vi "SubVI_counter_PM.VI"(2 "DeviceIndex":i32, 3 "Ch1 parameters":T1={"Ch1 Offs"=0, "Ch1 TRG Edge"=0, "Ch1 TRG Lvl"=-50} {"Ch1 TRG Lvl" min=-1200 max=1200 step=10; "Ch1 TRG Edge" min=0 max=1; "Ch1 Offs" min=-99999 max=99999 step=1}, 4 "Acq.Time (ms)":i32=10000 min=1 max=3600000 step=100) -> (0 "FiFoOverrun":bool, 1 "Counts":i32)   [LabVIEW 2013]
uses:
  th260lib.dll
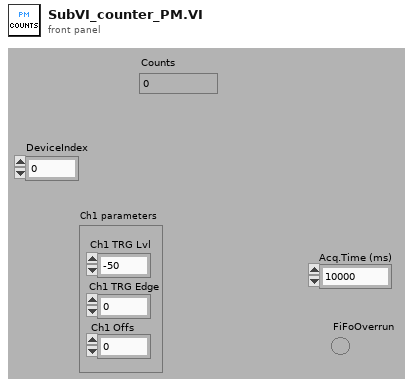
[diagram p1: front panel]
types:
  T1 = cluster{"Ch1 Offs":i32, "Ch1 TRG Edge":i32, "Ch1 TRG Lvl":i32}
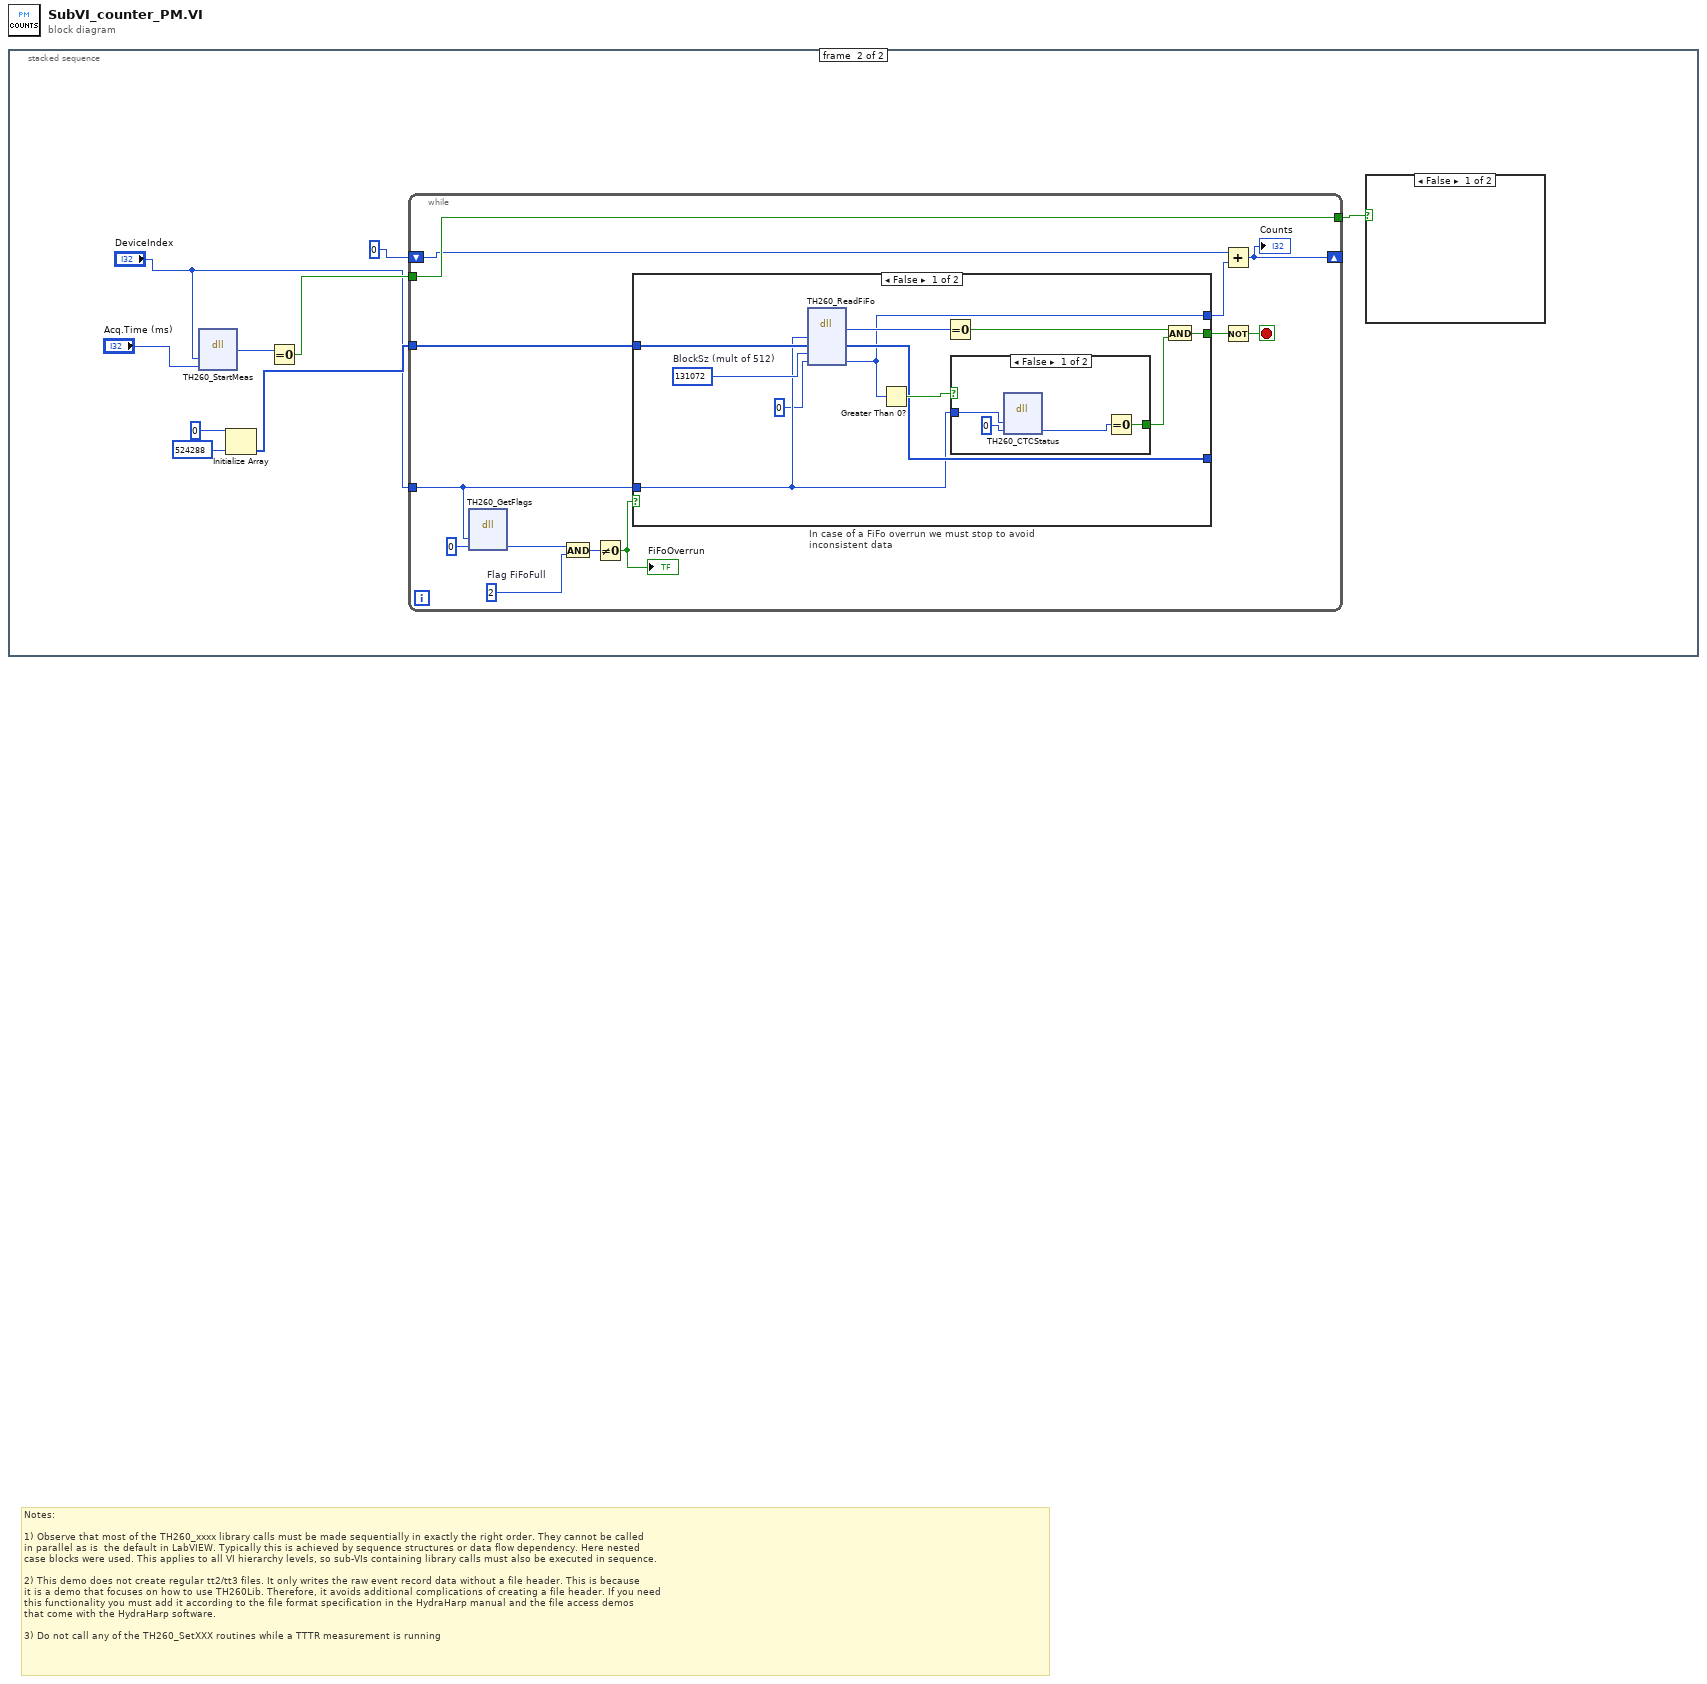
[diagram p0: block diagram]
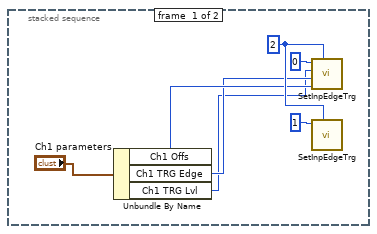
[diagram p2: hidden frame]
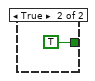
[diagram p3: hidden frame]
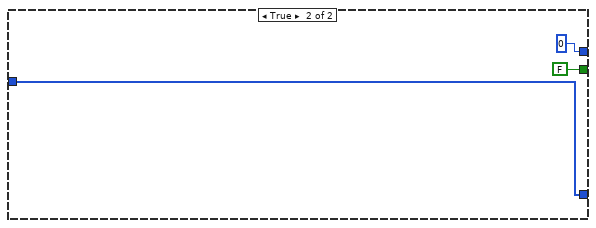
[diagram p4: hidden frame]
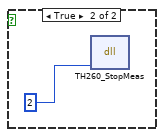
[diagram p5: hidden frame]
diagram:
  # "Notes: \n\n1) Observe that most of the TH260_xxxx library calls must be made sequentially in exactly the right order. They cannot be called \nin parallel as is  the default in LabVIEW. Typically this is achieved by sequence structures or data flow dependency. Here nested \ncase blocks were used. This applies to all VI hierarchy levels, so sub-VIs containing library calls must also be executed in sequence.\n\n2) This demo does not create regular tt2/tt3 files. It only writes the raw event record data without a file header. This is because \nit is a demo that focuses on how to use TH260Lib. Therefore, it avoids additional complications of creating a file header. If you need \nthis functionality you must add it according to the file format specification in the HydraHarp manual and the file access demos \nthat come with the HydraHarp software. \n\n3) Do not call any of the TH260_SetXXX routines while a TTTR measurement is running"
  n1 = stacked-sequence {
    frame #0 {
      w5 = 2 ("DeviceIndex")
      n2 = Unbundle By Name("Ch1 parameters") -> ("Ch1 Offs"=w3:i32, "Ch1 TRG Edge"=w2:i32, "Ch1 TRG Lvl"=w1:i32)
      n3 = call "SetInpEdgeTrg.vi"("Channel"=0, "CFD Level"=w1, "CFD ZeroX"=w2, "Offset"=w3, "DeviceIndex"=w5) -> ()  [unwired: 1 in, 1 out]
      n4 = call "SetInpEdgeTrg.vi"("Channel"=1, "DeviceIndex"=w5) -> ()  [unwired: 4 in, 1 out]
    }
    frame #1 {
      n5 = dll-call lib="th260lib.dll" fn="TH260_StartMeas"("devidx"="DeviceIndex", "tacq"="Acq.Time (ms)") -> (w14:i32)  [unwired: 5 in, 2 out]
      n6 = Initialize Array(u8 0, 524288) -> (w13:u8[])
      n7 = Equal To 0?(x=w14) -> (x = 0?=w15:bool)
      n8 = while {
        tunnel: w15 -> [w29]
        tunnel: [w29] -> w10
        shift-right: [w28] -> _
        shift-left: 0 -> [w17]
        tunnel: w13 -> [w22]
        tunnel: "DeviceIndex" -> [w23]
        stop <- w19 stop-if-true
        w27 = 2  # Flag FiFoFull
        n9 = dll-call lib="th260lib.dll" fn="TH260_GetFlags"("devidx"=w23, "flags"=0) -> ("flags"=w24:i32)  [unwired: 5 in, 2 out]
        n10 = And(x=w24, y=w27) -> (x .and. y?=w26:i32)
        n11 = Not Equal To 0?(x=w26) -> (x != 0?=w21:bool)
        "FiFoOverrun" <- w21
        n12 = case "In case of a FiFo overrun we must stop to avoid inconsistent data" shown="False" w21 {
          tunnel: w22 -> [w38 w47]
          tunnel: [w32 0] -> w18
          tunnel: [w37 w47] -> _
          tunnel: [w39 FALSE] -> w20
          tunnel: w23 -> [w35 _]
          frame False {
            w36 = 131072  # BlockSz (mult of 512)
            n13 = dll-call lib="th260lib.dll" fn="TH260_ReadFiFo"("devidx"=w35, "buffer"=w38, "blocksize"=w36, "nactual"=0) -> (w33:i32, "buffer"=w37:u8[], "nactual"=w32:i32)  [unwired: 5 in, 2 out]
            n14 = Greater Than 0?(x=w32) -> (x > 0?=w40:bool)
            n15 = Equal To 0?(x=w33) -> (x = 0?=w31:bool)
            n16 = case shown="False" w40 {
              tunnel: [w44 TRUE] -> w30
              tunnel: w35 -> [w43 _]
              frame False {
                n17 = dll-call lib="th260lib.dll" fn="TH260_CTCStatus"("devidx"=w43, "status"=0) -> ("status"=w41:i32)  [unwired: 5 in, 2 out]
                n18 = Equal To 0?(x=w41) -> (x = 0?=w44:bool)
              }
              frame True {
              }
            }
            n19 = And(x=w31, y=w30) -> (x .and. y?=w39:bool)
          }
          frame True {
          }
        }
        n20 = Add(x=w17, y=w18) -> (x+y=w28:i32)
        "Counts" <- w28
        n21 = Not(x=w20) -> (.not. x?=w19:bool)
      }
      n22 = case shown="False" w10 {
        frame False {
        }
        frame True {
          n23 = dll-call lib="th260lib.dll" fn="TH260_StopMeas"("devidx"=2) -> ()  [unwired: 5 in, 2 out]
        }
      }
    }
  }
